vi "Acquire Node Information.vi"(8 "error in (no error)":errorcluster, 9 "Activate Cell(True)":bool=TRUE, 10 "Node Tag":string, 11 "TREE in":refnum<class "MyTreeAPI.lvclass">) -> (0 "error out":errorcluster, 2 "Node Hierachy":string[](array[string]), 3 "TREE out":refnum<class "MyTreeAPI.lvclass">)   [LabVIEW 2015, in "MyTreeAPI.lvclass"]
uses:
  MyTreeAPI.lvclass
  MyTreeAPI.lvclass/MyTreeAPI.ctl
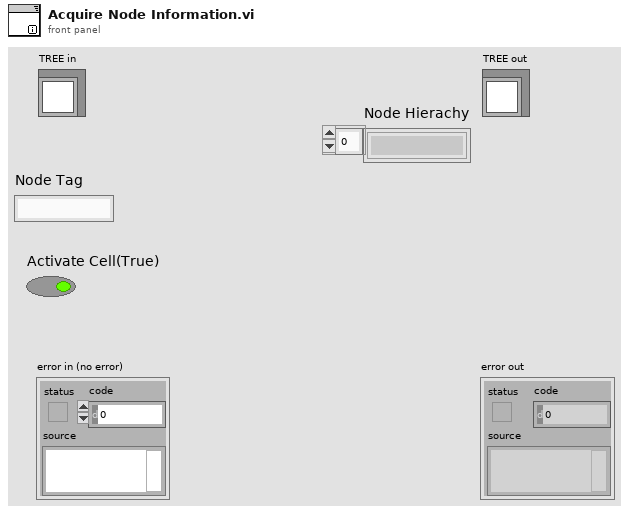
[diagram p1: front panel]
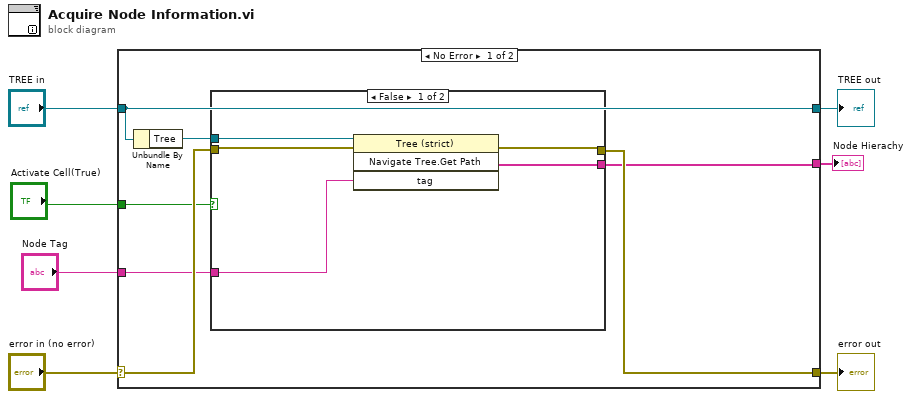
[diagram p0: block diagram]
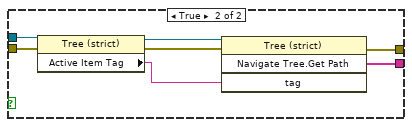
[diagram p2: hidden frame]
diagram:
  n1 = case shown="No Error" "error in (no error)" {
    selector: "error in (no error)" -> [w10 w28]
    tunnel: [w13 w28] -> w6
    tunnel: [w14 w27] -> w4
    tunnel: "TREE in" -> [w14 w27]
    tunnel: [w12 _] -> w3
    tunnel: "Activate Cell(True)" -> [w9 _]
    tunnel: "Node Tag" -> [w8 _]
    frame No Error {
      n2 = Unbundle By Name(w14) -> ("Tree"=w11:refnum<vi>)
      n3 = case shown="False" w9 {
        tunnel: [w17 w26] -> w13
        tunnel: [w16 w25] -> w12
        tunnel: w11 -> [w19 w24]
        tunnel: w10 -> [w18 w23]
        tunnel: w8 -> [w15 _]
        frame False {
          n4 = invoke class="Tree (strict)" method="Navigate Tree.Get Path"(reference=w19, error in=w18, "tag"=w15) -> (error out=w17:errorcluster, "Navigate Tree:Get Path"=w16:string[])  [unwired: 1 in, 2 out]
        }
        frame True {
          n5 = property class="Tree (strict)"(reference=w24, error in=w23) -> (reference out=w21:refnum<vi>, error out=w20:errorcluster, "Active Item Tag"=w22:string)
          n6 = invoke class="Tree (strict)" method="Navigate Tree.Get Path"(reference=w21, error in=w20, "tag"=w22) -> (error out=w26:errorcluster, "Navigate Tree:Get Path"=w25:string[])  [unwired: 1 in, 2 out]
        }
      }
    }
    frame Error {
    }
  }
  "error out" <- w6
  "TREE out" <- w4
  "Node Hierachy" <- w3
